vi "CIAdjustBeadPos.vi"(9 "Corner-based bead pos":cluster{"X":i32, "Y":i32}[](array[cluster]), 11 "Camera state":variant) -> (1 "Adjusted bead pos (out)":cluster{"X":i32, "Y":i32}[](array[cluster]), 3 "Camera state (out)":variant)   [LabVIEW 2011]
uses:
  mkCameraData.ctl
  CameraConfig.ctl
  Main/Camera/GenericCameraConfigType.ctl
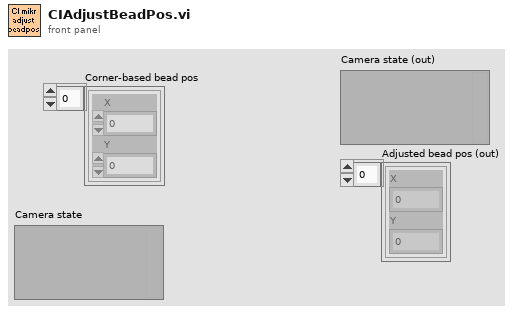
[diagram p1: front panel]
types:
  T1 = typedef "CameraConfig.ctl" = cluster{"Gain [1-4]":sgl, "Offset":i16, "Mode":i16, "ROIs":cluster{"X":i32, "Y":i32}[], "ROI Size":cluster{"X":i32, "Y":i32}, "Number of buffers":i32, "Use hardware multiple-ROI?":bool, "GenericCameraConfig":T2}
  T2 = typedef "GenericCameraConfigType.ctl" = cluster{"Framerate (Hz)":i32, "Exposure time (us)":i32, "Image size":cluster{"Width":i32, "Height":i32}, "Number of buffers":i32}
  T3 = typedef "mkCameraData.ctl" = cluster{"Session":refnum<k11>, "Settings":T1}
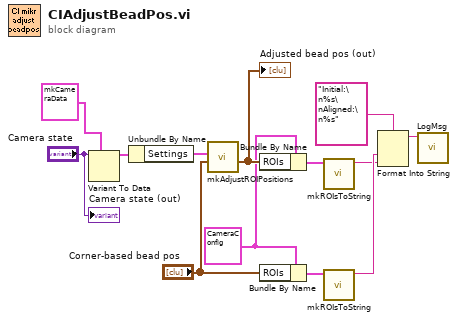
[diagram p0: block diagram]
diagram:
  w7 = T1 {"Gain [1-4]"=1.0, "Offset"=50, "Mode"=6, "ROIs"=[], "ROI Size"={"X"=0, "Y"=0}, "Number of buffers"=40, "Use hardware multiple-ROI?"=TRUE, "GenericCameraConfig"={"Framerate (Hz)"=60, "Exposure time (us)"=5000, "Image size"={"Width"=1280, "Height"=1024}, "Number of buffers"=0}} ("Settings")
  n1 = Variant To Data(type=T3 {"Session"=refnum, "Settings"={"Gain [1-4]"=1.0, "Offset"=50, "Mode"=6, "ROIs"=[], "ROI Size"={"X"=0, "Y"=0}, "Number of buffers"=40, "Use hardware multiple-ROI?"=TRUE, "GenericCameraConfig"={"Framerate (Hz)"=60, "Exposure time (us)"=5000, "Image size"={"Width"=1280, "Height"=1024}, "Number of buffers"=0}}} ("Camera settings"), Variant="Camera state") -> (data=w11:T3)  [unwired: 1 in, 1 out]
  n2 = Unbundle By Name(w11) -> ("Settings"=w10:T1)
  n3 = call "mkAdjustROIPositions.vi"("Corner-based bead pos"="Corner-based bead pos", "Camera settings"=w10) -> ("Adjusted bead pos (out)"=w8:cluster{"X":i32, "Y":i32}[])  [unwired: 9 in]
  "Adjusted bead pos (out)" <- w8
  n4 = Bundle By Name(cluster=w7, "ROIs"=w8) -> (w5:T1)
  n5 = Bundle By Name(cluster=w7, "ROIs"="Corner-based bead pos") -> (w4:T1)
  n6 = call "mkROIsToString.vi"("Settings"=w5) -> ("ROIs description"=w2:string)  [unwired: 10 in]
  n7 = call "mkROIsToString.vi"("Settings"=w4) -> ("ROIs description"=w3:string)  [unwired: 10 in]
  n8 = Format Into String(format string="Initial:\n%s\nAligned:\n%s", w3, w2) -> (resulting string=w1:string)  [unwired: 2 in, 1 out]
  n9 = call "LogMsg.vi"("msg"=w1) -> ()  [unwired: 11 in]
  "Camera state (out)" <- "Camera state"
